vi "Measurement UI.vi"() -> ()   [LabVIEW 2021, in "Arbitrary Mode_PMIC UI.lvlib"]
uses:
  Arbitrary Mode_PMIC UI.lvlib
panel:
  in  "MeasGraphs":T1(tab)
  out "SourceVoltageV/STimeGraph":waveform(dbl)(graph) caption="Load Transient"
  in  "SourceOutput Voltage v/s Time":string="SOURCE VOLTAGE vs TIME"
  out "OutputVoltageV/STimeGraph":waveform(dbl)(graph) caption="Load Transient"
  in  "LoadOutput Voltage v/s Time":string="LOAD VOLTAGE vs TIME"
  out "ScopeAmplitudeV/STime":waveform(dbl)(graph) caption="Load Transient"
  in  "ScopeOutput Voltage v/s Time":string="SCOPE AMPLITUDE vs TIME"
  out "Scope amplitude dt":dbl
  out "Scope amplitudes":dbl[](array[numeric])
  out "Load voltages":dbl[](array[numeric])
  out "Load voltage dt":dbl
  out "Source voltages":dbl[](array[numeric])
  out "Source voltage dt":dbl
  in  "Load resource name":string
  in  "Scope resource name":string
  in  "Source resource name":string
  in  "Source transient response":i32(ring)=1042 items=["Slow"=1041, "Normal"=1038, "Fast"=1039, "Custom"=1042]
  in  "MeasConfigurations":T2(tab)=enum."Load Config"
  in  "Source signal logging loop count":i64=1 caption="DATA LOGGING LOOP COUNT"
  in  "Source signal logging":u32[](array[ring]) caption="SIGNAL LOGGING" items=["Trapezoid", "Ramp"]
  in  "Source signal configuration":enum32{"Trapezoid Config", "Ramp Config"}(tab) caption="SIGNAL CONFIGURATION"
  in  "Trapezoid enable/disable":bool=TRUE caption="Trapezoid Enable/Disable"
  in  "Trapezoid voltage delay t2":dbl=0.005 caption="DELAY T2" format="%#_6ps"
  in  "Trapezoid voltage delay t1":dbl=0.005 caption="DELAY T1" format="%#_6ps"
  in  "Trapezoid voltatge pulse duration":dbl=0.005 caption="PULSE DURATION" format="%#_6ps"
  in  "Trapezoid voltage falling slew rate":dbl=50000.0 caption="VOLTAGE RISING SLEW RATE" format="%#_6pV/s"
  in  "Trapezoid voltage rising slew rate":dbl=50000.0 caption="VOLTAGE FALLING SLEW RATE" format="%#_6pV/s"
  in  "Trapezoid voltage set point 2(V2)":dbl=20.0 caption="VOLTAGE SET POINT 2" format="%#_6pV"
  in  "Trapezoid voltage set point 1(V1)":dbl=7.0 caption="VOLTAGE SET POINT 1" format="%#_6pV"
  in  "Ramp enable/disable":bool caption="Ramp Enable/Disable"
  in  "Ramp voltatge V2 time":dbl=0.005 caption="TIME for V1" format="%#_6ps"
  in  "Ramp voltage V1 time":dbl=0.005 caption="TIME for V1" format="%#_6ps"
  in  "Ramp voltage ramp rate":dbl=50000.0 caption="VOLTAGE RAMP RATE" format="%#_6pV/s"
  in  "Ramp voltage set point 2(V2)":dbl=20.0 caption="RAMP STOP VOLTAGE(V2)" format="%#_6pV"
  in  "Ramp voltage set point 1(V1)":dbl=0.1 caption="RAMP START VOLTAGE(V1)" format="%#_6pV"
  in  "Source sense":i32(ring)=1009 caption="SENSE" items=["Local"=1008, "Remote"=1009]
  in  "Source maximum power":dbl=300.0 caption="MAXIMUM POWER" format="%#_6pW"
  in  "Source current limit":dbl=0.25 caption="CURRENT LIMIT" format="%#_6pA"
  in  "Source set-up voltage":dbl=8.0 caption="SET VOLTAGE" format="%#_6pV"
  in  "PPSResourceName":refnum<k15> caption="RESOURCE NAME"
  in  "Source voltage pole-zero ratio":dbl=2.0 caption="POLE-ZERO RATIO"
  in  "Source voltage gain bandwidth":dbl=2000.0 caption="GAIN BANDWIDTH" format="%#_6pHz"
  in  "Source voltage compensation frequency":dbl=3530.0 caption="COMP. FREQUENCY" format="%#_6pHz"
  in  "Source fast":bool
  in  "Source normal":bool
  in  "Source slow":bool
  in  "Source SourceAdapt":string="Voltage SourceAdapt Parameters"
  in  "Source sample rate":dbl=1800000.0 caption="SAMPLE RATE" format="%#_6pS/s"
  in  "Load current level range":dbl=4.0 caption="CURRENT LEVEL RANGE" format="%#_6pA"
  in  "Load sense":i32(ring)=1009 caption="SENSE" items=["Local"=1008, "Remote"=1009]
  in  "ELOADResourceName":refnum<k15> caption="RESOURCE NAME"
  in  "Load current level":dbl=1.0 caption="CURRENT  LEVEL" format="%#_6pA"
  in  "Load voltage limit range":dbl=6.0 caption="VOLTAGE LIMIT RANGE" format="%#_6pV"
  in  "Load enable/disable":bool caption="Load Enable/Disable"
  out "Load status":string="Load is disabled"
  in  "Scope vertical range":dbl=10.0 caption="VERTICAL RANGE"
  out "Scope status":string="Scope is disabled"
  in  "Scope enable/disable":bool caption="Scope Enable/Disable"
  in  "SCOPEResourceName":refnum<k15> caption="RESOURCE NAME"
  in  "Scope probe attenuation":dbl=1.0 caption="PROBE ATTENUATION"
  in  "Scope sample rate":dbl=1800000.0 caption="SAMPLE RATE" format="%#_6pHz"
  in  "Scope output channel name":string="0" caption="INPUT CHANNEL NAME"
  in  "Scope vertical coupling":enum32{"AC", "DC"}(ring)=enum."DC" caption="VERTICAL COUPLING"
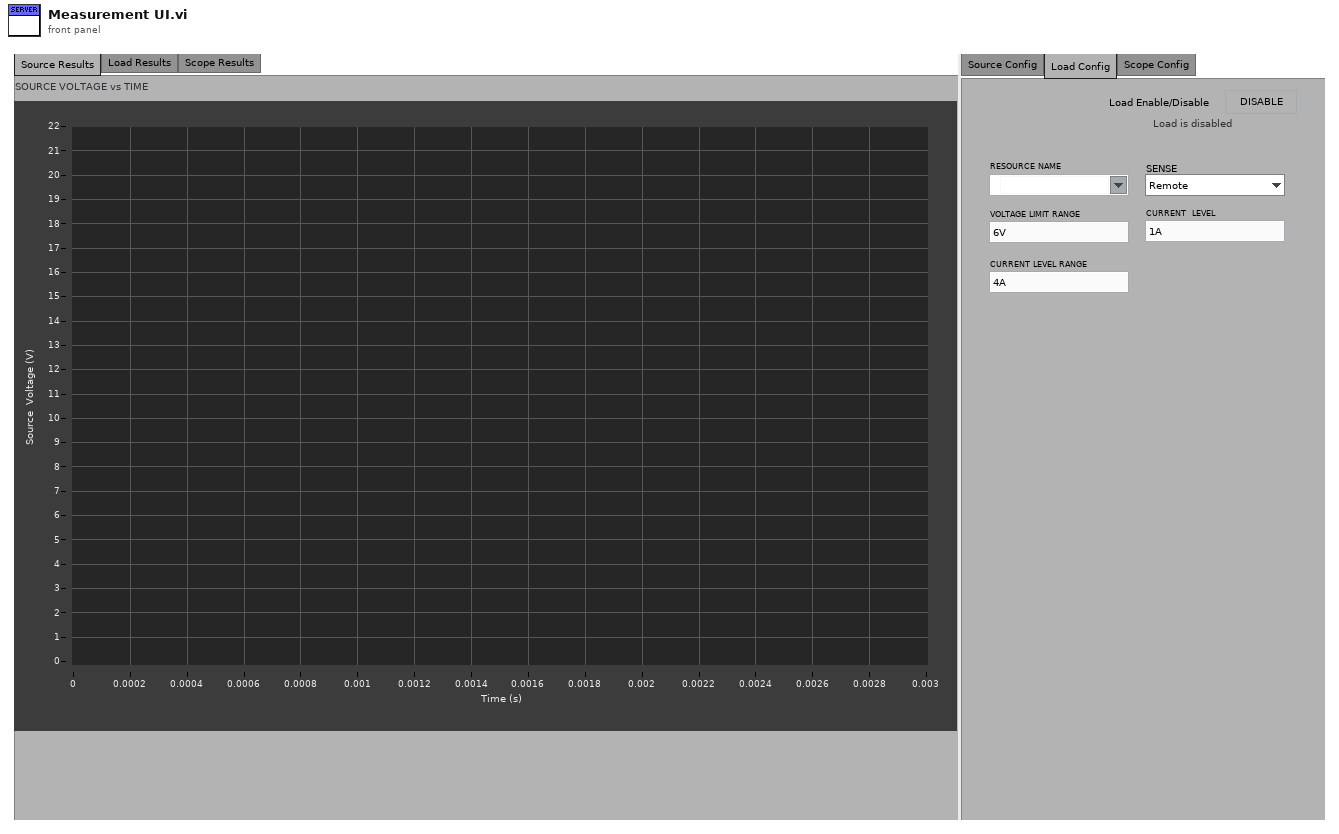
[diagram p1: front panel]
types:
  T1 = enum32{"Source Results", "Load Results", "Scope Results", "Hidden Controls"}
  T2 = enum32{"Source Config", "Load Config", "Scope Config"}
  T3 = enum8{"Enabled", "Disabled", "Disabled and Grayed Out"}
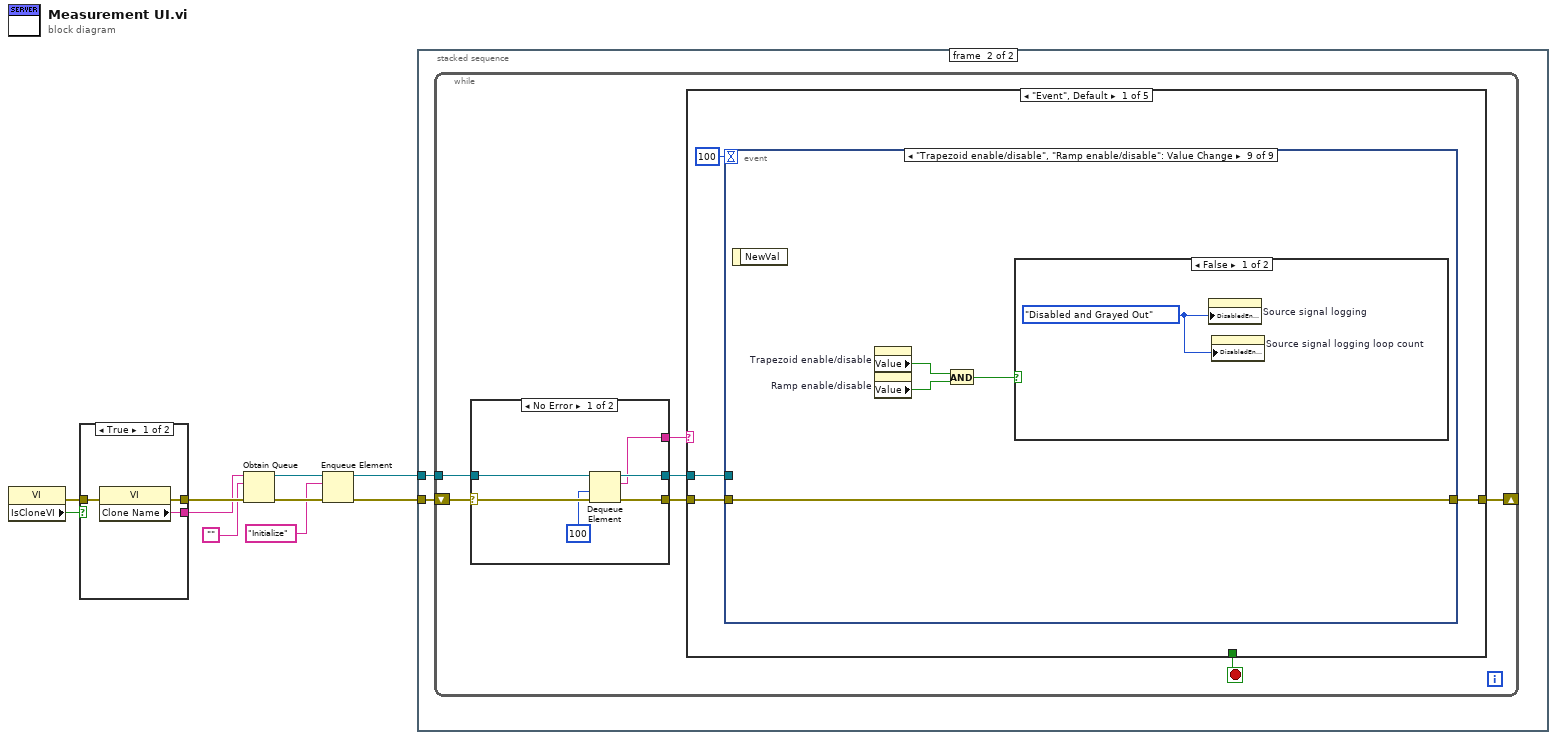
[diagram p0: block diagram]
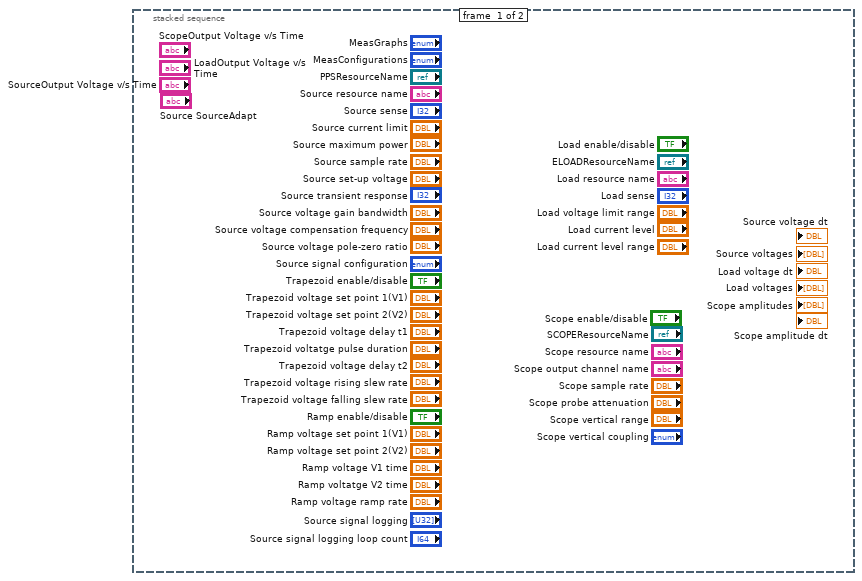
[diagram p2: hidden frame]
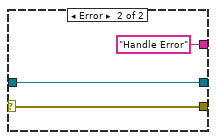
[diagram p3: hidden frame]
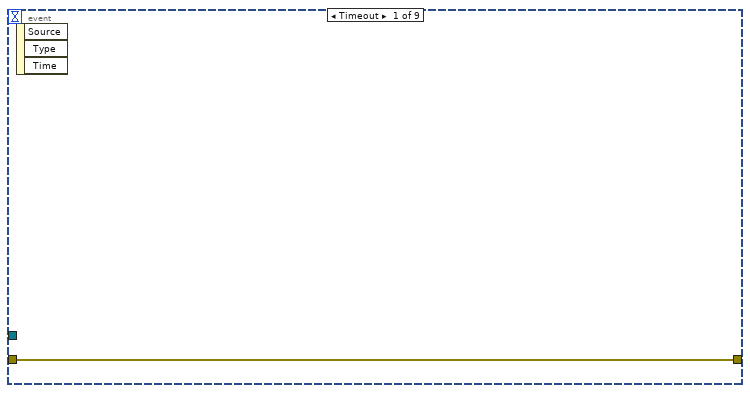
[diagram p4: hidden frame]
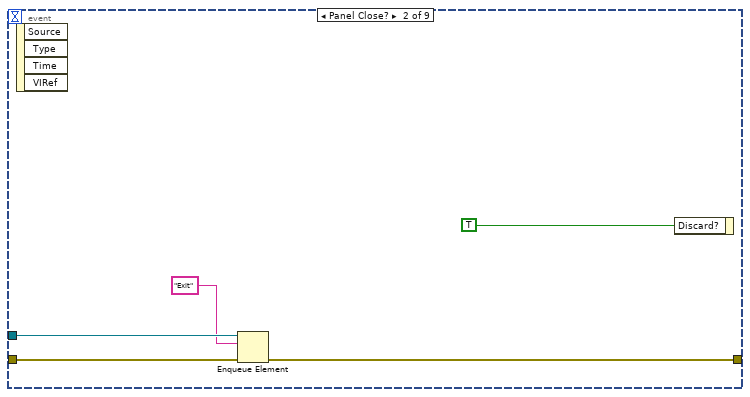
[diagram p5: hidden frame]
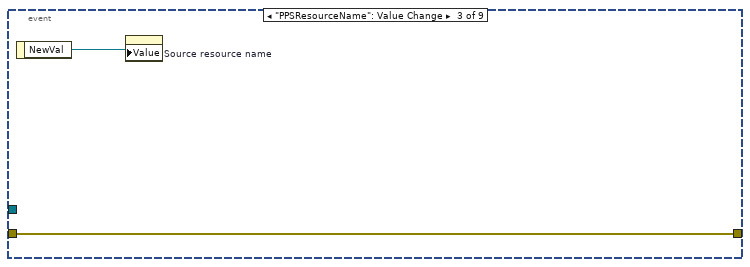
[diagram p6: hidden frame]
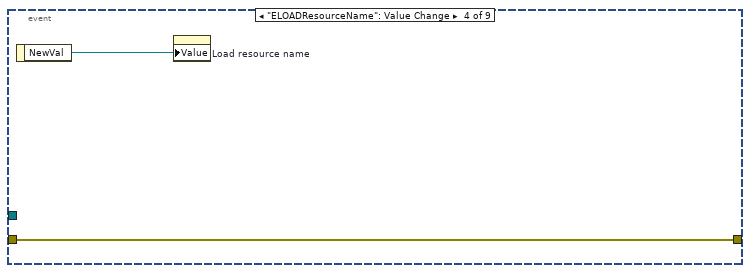
[diagram p7: hidden frame]
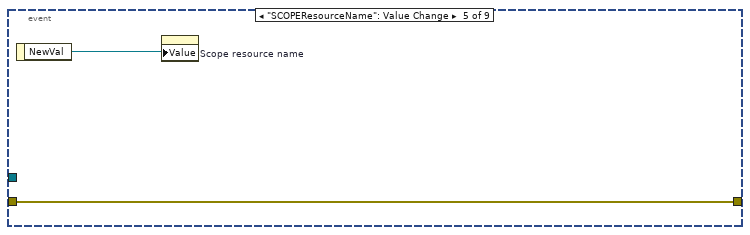
[diagram p8: hidden frame]
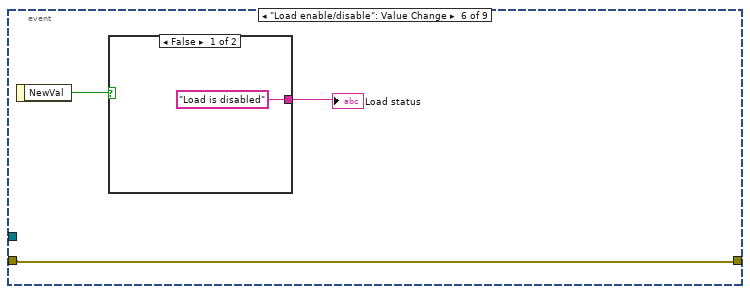
[diagram p9: hidden frame]
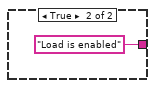
[diagram p10: hidden frame]
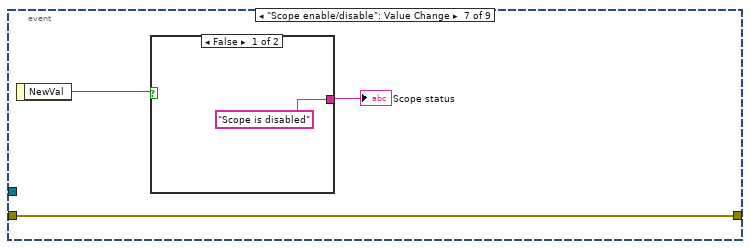
[diagram p11: hidden frame]
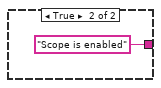
[diagram p12: hidden frame]
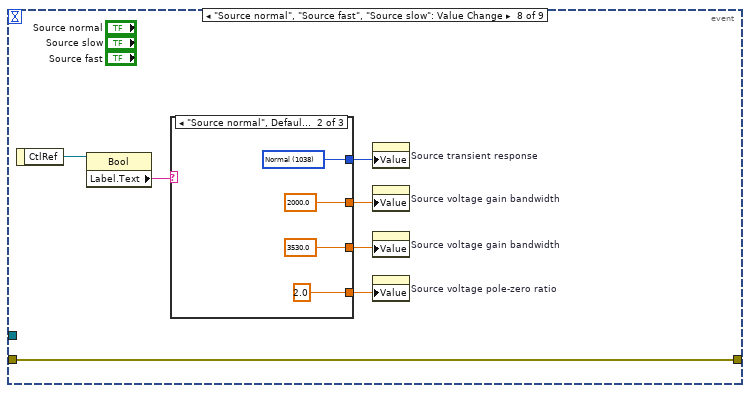
[diagram p13: hidden frame]
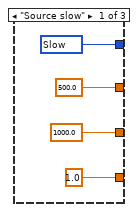
[diagram p14: hidden frame]
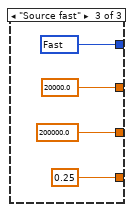
[diagram p15: hidden frame]
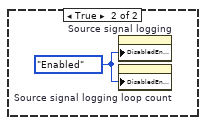
[diagram p16: hidden frame]
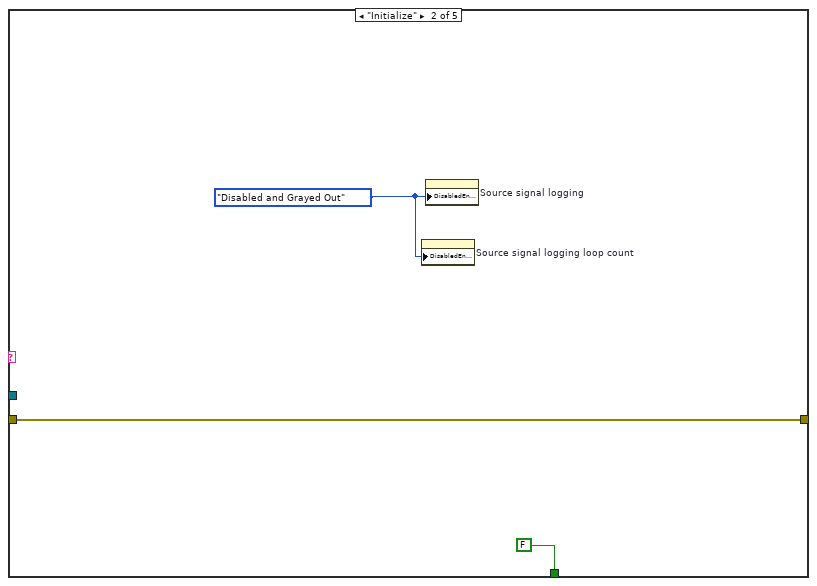
[diagram p17: hidden frame]
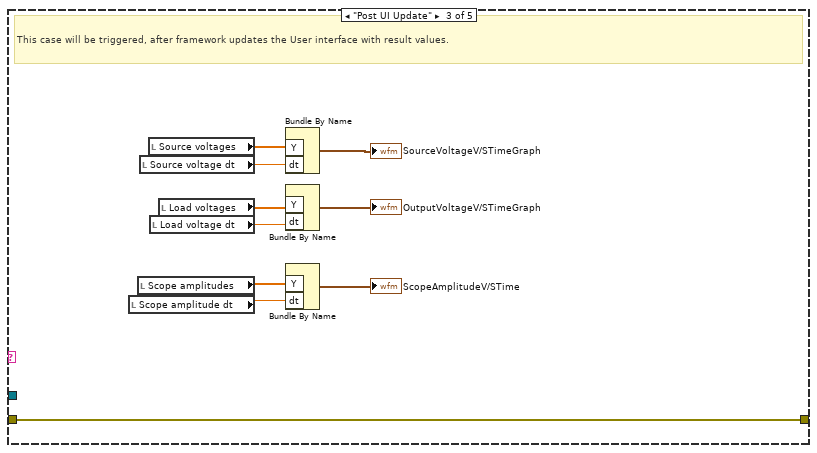
[diagram p18: hidden frame]
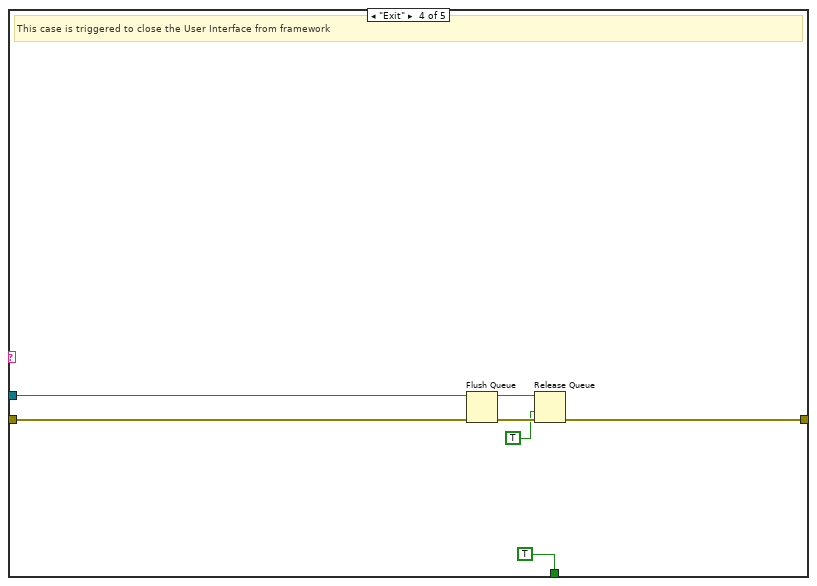
[diagram p19: hidden frame]
diagram:
  n1 = property class="VI"() -> (error out=w1:errorcluster, "IsCloneVI"=w2:bool)  [unwired: 2 in, 1 out]
  n2 = case shown="True" w2 {
    tunnel: [w13 w16] -> w10
    tunnel: [w12 w15] -> w9
    tunnel: w1 -> [w11 w14]
    frame True {
      n3 = property class="VI"(error in=w11) -> (error out=w13:errorcluster, "Clone Name"=w12:string)  [unwired: 1 in, 1 out]
    }
    frame False {
      n4 = property class="VI"(error in=w14) -> (error out=w16:errorcluster, "Name"=w15:string)  [unwired: 1 in, 1 out]
    }
  }
  n5 = Obtain Queue(name (unnamed)=w9, element data type="", error in (no error)=w10) -> (queue out=w6:refnum<queue>, error out=w8:errorcluster)  [unwired: 2 in, 1 out]
  n6 = Enqueue Element(queue=w6, element="Initialize", error in (no error)=w8) -> (queue out=w5:refnum<queue>, error out=w7:errorcluster)  [unwired: 1 in, 1 out]
  n7 = stacked-sequence {
    tunnel: w7 -> [_ w18]
    tunnel: w5 -> [_ w17]
    frame #0 {
    }
    frame #1 {
      n8 = while {
        shift-right: [w20] -> _
        shift-left: w18 -> [w25]
        tunnel: w17 -> [w23]
        stop <- w19 stop-if-true
        n9 = case shown="No Error" w25 {
          selector: w25 -> [w31 w34]
          tunnel: [w30 w34] -> w24
          tunnel: w23 -> [w29 w33]
          tunnel: [w28 w33] -> w22
          tunnel: [w27 "Handle Error"] -> w21
          frame No Error {
            n10 = Dequeue Element(queue=w29, timeout in ms (-1)=100, error in (no error)=w31) -> (queue out=w28:refnum<queue>, element=w27:string, error out=w30:errorcluster)  [unwired: 1 out]
          }
          frame Error {
          }
        }
        n11 = case shown="\"Event\", Default" w21 {
          tunnel: w24 -> [w37 w88 w98 w105 w106]
          tunnel: w22 -> [w35 _ _ w103 _]
          tunnel: [w38 w88 w98 w100 w106] -> w20
          tunnel: [_ FALSE _ TRUE _] -> w19
          frame "Event", Default {
            n12 = event shown="[8] \"Trapezoid enable/disable\", \"Ramp enable/disable\": Value Change" {
              selector: _ -> [_ _ _ _ _ _ _ _ _]
              dyn-events: _ -> [_ _ _ _ _ _ _ _ _]
              timeout: 100 -> [_ _ _ _ _ _ _ _ _]
              tunnel: [w39 w42 w45 w47 w49 w51 w56 w61 w80] -> w38
              tunnel: w37 -> [w39 w43 w45 w47 w49 w51 w56 w61 w80]
              tunnel: w35 -> [_ w41 _ _ _ _ _ _ _]
              event Timeout {
                n13 = event-data() -> ()  [unwired: 1 in, 3 out]
              }
              event Panel Close? {
                n14 = event-data() -> ()  [unwired: 1 in, 4 out]
                n15 = Enqueue Element(queue=w41, element="Exit", error in (no error)=w43) -> (error out=w42:errorcluster)  [unwired: 1 in, 2 out]
                n16 = event-data("Discard?"=TRUE) -> ()  [unwired: 1 in, 1 out]
              }
              event "PPSResourceName": Value Change {
                n17 = event-data() -> ("NewVal"=w46:refnum<k15>)  [unwired: 1 in]
                n18 = property on="Source resource name" class="Str"("Value"=w46) -> ()  [unwired: 2 in, 2 out]
              }
              event "ELOADResourceName": Value Change {
                n19 = event-data() -> ("NewVal"=w48:refnum<k15>)  [unwired: 1 in]
                n20 = property on="Load resource name" class="Str"("Value"=w48) -> ()  [unwired: 2 in, 2 out]
              }
              event "SCOPEResourceName": Value Change {
                n21 = event-data() -> ("NewVal"=w50:refnum<k15>)  [unwired: 1 in]
                n22 = property on="Scope resource name" class="Str"("Value"=w50) -> ()  [unwired: 2 in, 2 out]
              }
              event "Load enable/disable": Value Change {
                n23 = event-data() -> ("NewVal"=w53:bool)  [unwired: 1 in]
                n24 = case shown="False" w53 {
                  tunnel: ["Load is disabled" ("Load status") "Load is enabled" ("Load status")] -> w52
                  frame False {
                  }
                  frame True {
                  }
                }
                "Load status" <- w52
              }
              event "Scope enable/disable": Value Change {
                n25 = event-data() -> ("NewVal"=w58:bool)  [unwired: 1 in]
                n26 = case shown="False" w58 {
                  tunnel: ["Scope is disabled" ("Load status") "Scope is enabled" ("Load status")] -> w57
                  frame False {
                  }
                  frame True {
                  }
                }
                "Scope status" <- w57
              }
              event "Source normal", "Source fast", "Source slow": Value Change {
                n27 = event-data() -> ("CtlRef"=w62:refnum<vi>)  [unwired: 1 in]
                n28 = property class="Bool"(reference=w62) -> ("Label.Text"=w67:string)  [unwired: 1 in, 2 out]
                n29 = case shown="\"Source normal\", Default" w67 {
                  tunnel: [w71 w75 w79] -> w66
                  tunnel: [500.0 ("Source voltage gain bandwidth") 2000.0 ("Source voltage gain bandwidth") 20000.0 ("Source voltage gain bandwidth")] -> w65
                  tunnel: [1000.0 ("Source voltage compensation frequency") 3530.0 ("Source voltage compensation frequency") 200000.0 ("Source voltage compensation frequency")] -> w63
                  tunnel: [1.0 ("Source voltage pole-zero ratio") 2.0 ("Source voltage pole-zero ratio") 0.25 ("Source voltage pole-zero ratio")] -> w64
                  frame "Source slow" {
                    w71 = 1041 items=["Slow"=1041, "Normal"=1038, "Fast"=1039, "Custom"=1042] ("Source transient response")
                  }
                  frame "Source normal", Default {
                    w75 = 1038 items=["Slow"=1041, "Normal"=1038, "Fast"=1039, "Custom"=1042] ("Source transient response")
                  }
                  frame "Source fast" {
                    w79 = 1039 items=["Slow"=1041, "Normal"=1038, "Fast"=1039, "Custom"=1042] ("Source transient response")
                  }
                }
                n30 = property on="Source transient response" class="Ring (strict)"("Value"=w66) -> ()  [unwired: 2 in, 2 out]
                n31 = property on="Source voltage gain bandwidth" class="DigNum (strict)"("Value"=w65) -> ()  [unwired: 2 in, 2 out]
                n32 = property on="Source voltage gain bandwidth" class="DigNum (strict)"("Value"=w63) -> ()  [unwired: 2 in, 2 out]
                n33 = property on="Source voltage pole-zero ratio" class="DigNum (strict)"("Value"=w64) -> ()  [unwired: 2 in, 2 out]
              }
              event "Trapezoid enable/disable", "Ramp enable/disable": Value Change {
                n34 = event-data() -> ()  [unwired: 1 in, 1 out]
                n35 = property on="Trapezoid enable/disable" class="Bool (strict)"() -> ("Value"=w83:bool)  [unwired: 2 in, 2 out]
                n36 = property on="Ramp enable/disable" class="Bool (strict)"() -> ("Value"=w82:bool)  [unwired: 2 in, 2 out]
                n37 = And(x=w83, y=w82) -> (x .and. y?=w81:bool)
                n38 = case shown="False" w81 {
                  frame False {
                    w84 = T3."Disabled and Grayed Out" ("Disabled")
                    n39 = property on="Source signal logging" class="Arr (strict)"("DisabledEnum"=w84) -> ()  [unwired: 2 in, 2 out]
                    n40 = property on="Source signal logging loop count" class="DigNum (strict)"("DisabledEnum"=w84) -> ()  [unwired: 2 in, 2 out]
                  }
                  frame True {
                    w85 = T3."Enabled" ("Disabled")
                    n41 = property on="Source signal logging" class="Arr (strict)"("DisabledEnum"=w85) -> ()  [unwired: 2 in, 2 out]
                    n42 = property on="Source signal logging loop count" class="DigNum (strict)"("DisabledEnum"=w85) -> ()  [unwired: 2 in, 2 out]
                  }
                }
              }
            }
          }
          frame "Initialize" {
            w86 = T3."Disabled and Grayed Out" ("Disabled")
            n43 = property on="Source signal logging loop count" class="DigNum (strict)"("DisabledEnum"=w86) -> ()  [unwired: 2 in, 2 out]
            n44 = property on="Source signal logging" class="Arr (strict)"("DisabledEnum"=w86) -> ()  [unwired: 2 in, 2 out]
          }
          frame "Post UI Update" {
            # "This case will be triggered, after framework updates the User interface with result values."
            n45 = local read "Scope amplitude dt"() -> (w89:dbl)
            n46 = local read "Scope amplitudes"() -> (w90:dbl[])
            n47 = local read "Source voltage dt"() -> (w94:dbl)
            n48 = local read "Source voltages"() -> (w93:dbl[])
            n49 = local read "Load voltage dt"() -> (w91:dbl)
            n50 = local read "Load voltages"() -> (w92:dbl[])
            n51 = Bundle By Name("Y"=w93, "dt"=w94) -> (→"SourceVoltageV/STimeGraph":waveform(dbl))  [unwired: 1 in]
            n52 = Bundle By Name("Y"=w92, "dt"=w91) -> (→"OutputVoltageV/STimeGraph":waveform(dbl))  [unwired: 1 in]
            n53 = Bundle By Name("Y"=w90, "dt"=w89) -> (→"ScopeAmplitudeV/STime":waveform(dbl))  [unwired: 1 in]
          }
          frame "Exit" {
            # "This case is triggered to close the User Interface from framework"
            n54 = Flush Queue(queue=w103, error in (no error)=w105) -> (queue out=w102:refnum<queue>, error out=w101:errorcluster)  [unwired: 1 out]
            n55 = Release Queue(queue=w102, force destroy? (F)=TRUE, error in (no error)=w101) -> (error out=w100:errorcluster)  [unwired: 2 out]
          }
          frame "Handle Error" {
          }
        }
      }
    }
  }
